vi "Executable Set Logfile.vi"(8 "error in (no error)":errorcluster, 10 "relative Path":path, 11 "Build Spec Reference":refnum<vi>) -> (0 "error out":errorcluster, 3 "Build Spec Reference Dup":refnum<vi>)   [LabVIEW 2016, in "LabVIEW Project API__icon_lib_labview_project_api.lvlib"]
doc: "Returns a Build Specification Executable Version [Major, Minor, Fix, Build]\n\n<b>Author:</b> JG\n\n<b>ICON Technologies Pty Ltd</b>\nCopyright (C) 1990-2009\nAll Rights Reserved"
uses:
  LabVIEW Project API__icon_lib_labview_project_api.lvlib
panel:
  # "Output"
  # "Input"
  # "ICON Technologies Pty Ltd\nCopyright (C) 1990-2009\nAll Rights Reserved"
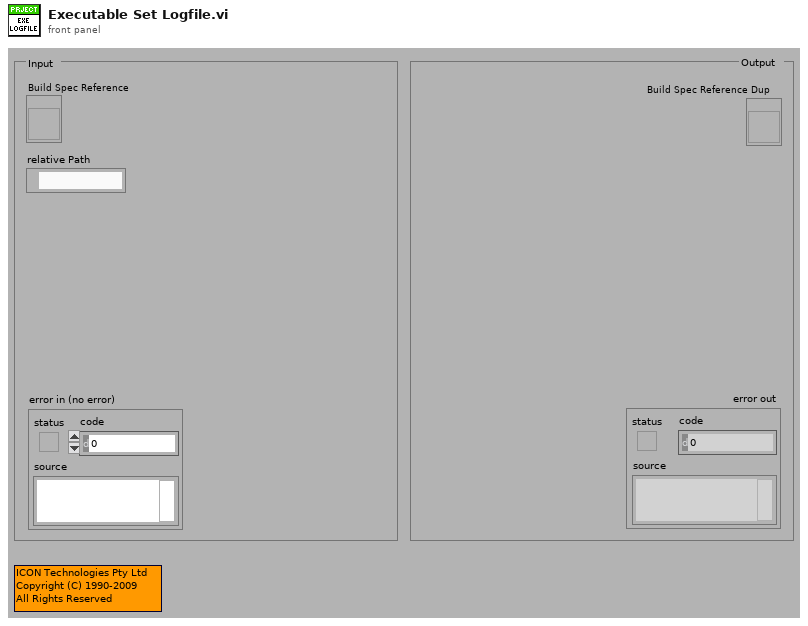
[diagram p1: front panel]
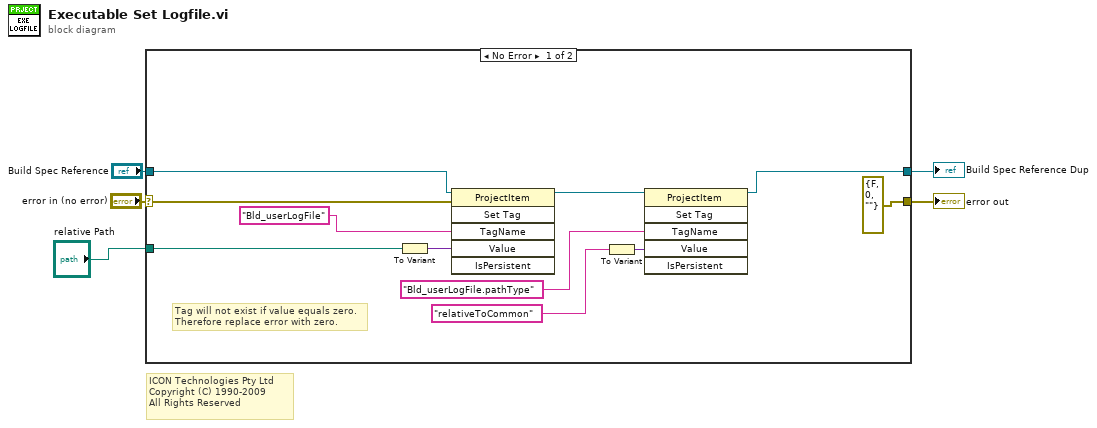
[diagram p0: block diagram]
diagram:
  # "ICON Technologies Pty Ltd\nCopyright (C) 1990-2009\nAll Rights Reserved"
  n1 = case shown="No Error" "error in (no error)" {
    selector: "error in (no error)" -> [w14 w18]
    tunnel: [errorcluster {"status"=FALSE, "code"=0, "source"=""} ("error out") w18] -> w4
    tunnel: "Build Spec Reference" -> [w15 w17]
    tunnel: [w9 w17] -> w2
    tunnel: "relative Path" -> [w11 _]
    frame No Error {
      # "Tag will not exist if value equals zero.\nTherefore replace error with zero."
      n2 = To Variant(anything=w11) -> (Variant=w12:variant)
      n3 = invoke class="ProjectItem" method="Set Tag"(reference=w15, error in=w14, "TagName"="Bld_userLogFile" ("Tag Name"), "Value"=w12) -> (reference out=w10:refnum<vi>)  [unwired: 2 in, 5 out]
      n4 = To Variant(anything="relativeToCommon" ("Tag Name")) -> (Variant=w7:variant)
      n5 = invoke class="ProjectItem" method="Set Tag"(reference=w10, "TagName"="Bld_userLogFile.pathType" ("Tag Name"), "Value"=w7) -> (reference out=w9:refnum<vi>)  [unwired: 3 in, 5 out]
    }
    frame Error {
    }
  }
  "error out" <- w4
  "Build Spec Reference Dup" <- w2
